vi "Add Calculation Name to Available Calculations Field.vi"(8 "error in (no error)":errorcluster, 10 "Device Item Ref":T1=18446744073709551615 format="%.0x", 11 "WaveformCalculation in":refnum<class "WaveformCalculation.lvclass">) -> (0 "error out":errorcluster, 3 "WaveformCalculation out":refnum<class "WaveformCalculation.lvclass">)   [LabVIEW 2015, in "WaveformCalculation.lvclass"]
uses:
  WaveformCalculation.lvclass
  <vilib>/NI Veristand/Custom Device API/Custom Device Item Ref.ctl
  WaveformCalculation.lvclass/WaveformCalculation.ctl
  Shared/Constants.vi
  <vilib>/NI Veristand/Custom Device API/Get Item Property (String Array).vi
  <vilib>/NI Veristand/Custom Device API/Set Item Property (String Array).vi
  <vilib>/NI VeriStand/Custom Device API/Custom Device API.lvlib
  Shared/Waveform-Processing-Custom-Device Shared.lvlib
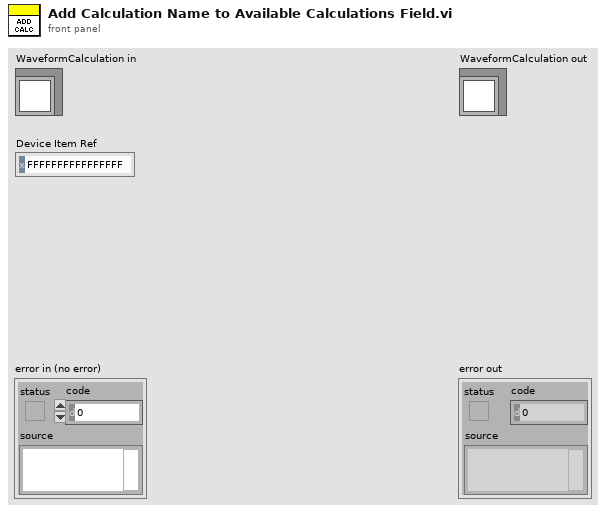
[diagram p1: front panel]
types:
  T1 = typedef "Custom Device API.lvlib/Custom Device Item Ref.ctl" = u64
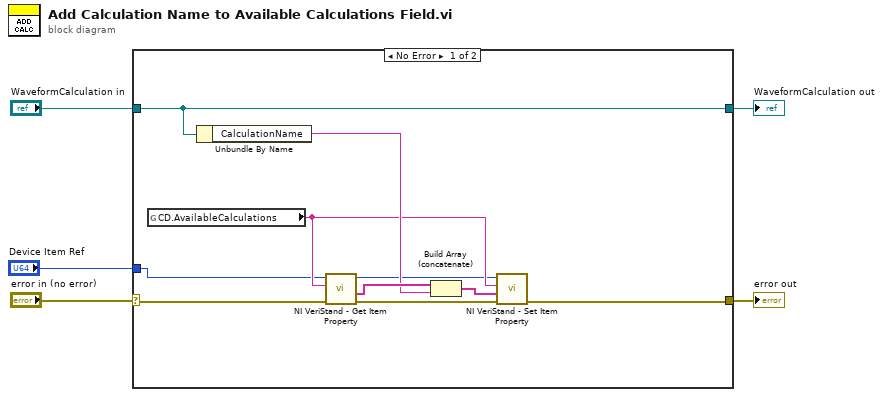
[diagram p0: block diagram]
diagram:
  n1 = case shown="No Error" "error in (no error)" {
    selector: "error in (no error)" -> [w12 w17]
    tunnel: [w14 w17] -> w4
    tunnel: [w15 w16] -> w2
    tunnel: "WaveformCalculation in" -> [w15 w16]
    tunnel: "Device Item Ref" -> [w7 _]
    frame No Error {
      n2 = global read "Constants.vi" "CD.AvailableCalculations"() -> (w8:string)
      n3 = Unbundle By Name(w15) -> ("CalculationName"=w10:string)
      n4 = call-poly <vilib>:"NI VeriStand - Get Item Property.vi"("error in (no error)"=w12, "Property Name"=w8, "Item Ref in"=w7) -> ("error out"=w13:errorcluster, "Value"=w11:string[], "Item Ref out"=w6:T1)  [unwired: 5 in, 1 out]
      n5 = Build Array (concatenate)(w11, w10) -> (w9:string[])
      n6 = call-poly <vilib>:"NI VeriStand - Set Item Property.vi"("error in (no error)"=w13, "Value"=w9, "Property Name"=w8, "Item Ref in"=w6) -> ("error out"=w14:errorcluster)  [unwired: 5 in, 2 out]
    }
    frame Error {
    }
  }
  "error out" <- w4
  "WaveformCalculation out" <- w2
